vi "MGCC_StaEst_error_cal.vi"(8 "f_MGCC_StaEst_An":dbl[][](array[numeric]), 9 "f_MGCC_StaEst_Vn":dbl[][](array[numeric]), 10 "cluster":T1) -> (0 "output_An":dbl[][](array[numeric]), 1 "Ang Err":dbl[][](array[numeric]), 2 "Mag Err":dbl[][](array[numeric]), 3 "output_Vn":dbl[][](array[numeric]))   [LabVIEW 2016]
uses:
  MGCC_StaEst_global.vi
  Model Management/Global_MdlMgmt.vi
  Finite State Machine/Sub-VIs/MGCC_FntStaMach_gobal.vi
  <vilib>/imath/engines/lvmath2/RunTimeEngine/IndexRead/NIMS M(S,$).vi
  <instcachedir>/0/NIMS M(S,$)_F24F360562DE41D8BE234322A2E15C65.lvgen/NIMS M(S,$)_F24F360562DE41D8BE234322A2E15C65_000.vi
  <vilib>/imath/engines/lvmath2/RunTimeEngine/BuiltInFunctions/length/NIMS_length(GV).vi
  <instcachedir>/0/NIMS_length(GV)_08A3D13377FD4E4B96F5795FBF3698FA.lvgen/NIMS_length(GV)_08A3D13377FD4E4B96F5795FBF3698FA_000.vi
  <vilib>/imathl/engines/lvmath/Functions/Error Handling/Create Error.vi
  <vilib>/imath/engines/lvmath2/RunTimeEngine/RangeToken/NIMS_Range_R3 - Integer.vi
  <instcachedir>/0/NIMS_Range_R3 - Integer_A435E2FF893B4C718FD5055FE39FE2F6.lvgen/NIMS_Range_R3 - Integer_A435E2FF893B4C718FD5055FE39FE2F6_000.vi
  <vilib>/imath/engines/lvmath2/RunTimeEngine/CommandStatement/MC_CommandStatement_break.vi
  <vilib>/imath/engines/lvmath2/RunTimeEngine/IndexRead/NIMS M($,S).vi
  <instcachedir>/0/NIMS M($,S)_3E5749BBB62E49528D4765A77F1F6D98.lvgen/NIMS M($,S)_3E5749BBB62E49528D4765A77F1F6D98_000.vi
  <vilib>/imath/engines/lvmath2/RunTimeEngine/IndexRead/NIMS V(S).vi
  <instcachedir>/0/NIMS V(S)_0488751826AF41519A22953C041130DC.lvgen/NIMS V(S)_0488751826AF41519A22953C041130DC_000.vi
  <vilib>/imath/engines/lvmath2/RunTimeEngine/IndexReplace/NIMS M(S,S)=S.vi
  <instcachedir>/0/NIMS M(S,S)=S_98E40400474E4398B113AE20298B4F82.lvgen/NIMS M(S,S)=S_98E40400474E4398B113AE20298B4F82_000.vi
  <vilib>/imath/engines/lvmath2/RunTimeEngine/IndexRead/NIMS M(S,S).vi
  <instcachedir>/0/NIMS M(S,S)_AC51E74150A542F7991B9634C66F3096.lvgen/NIMS M(S,S)_AC51E74150A542F7991B9634C66F3096_000.vi
  <vilib>/imath/engines/lvmath2/RunTimeEngine/ErrorHandling/NIMS_Create Error From Enums.vi
  <vilib>/imath/engines/lvmath2/RunTimeSupport/NIMS_Error if Not Equal.vi
  <instcachedir>/0/NIMS_Error if Not Equal_43252A79AD05436189442EC0C5E5AB8A.lvgen/NIMS_Error if Not Equal_43252A79AD05436189442EC0C5E5AB8A_000.vi
  <vilib>/imath/engines/lvmath2/RunTimeEngine/IndexRead/NIMS M(S).vi
  <instcachedir>/0/NIMS M(S)_B826C018497E4940AE96BD27B540B6FB.lvgen/NIMS M(S)_B826C018497E4940AE96BD27B540B6FB_000.vi
  <vilib>/imath/engines/lvmath2/RunTimeEngine/IndexReplace/NIMS M(S,$)=V.vi
  <instcachedir>/0/NIMS M(S,$)=V_BCCFA522A894489B8FA760383D74A164.lvgen/NIMS M(S,$)=V_BCCFA522A894489B8FA760383D74A164_000.vi
  <vilib>/imath/engines/lvmath2/RunTimeEngine/NodeEndStatement/NIMS_NodeEndStatement_Output.vi
  <instcachedir>/0/NIMS_NodeEndStatement_Output_53EC0D466D134D7ABD903AC30B43404B.lvgen/NIMS_NodeEndStatement_Output_53EC0D466D134D7ABD903AC30B43404B_002.vi
  <vilib>/imath/engines/lvmath2/RunTimeEngine/ErrorHandling/NIMS_Finalize Error.vi
panel:
  out "array w/ subset deleted":dbl[](array[numeric])
  out "error out":errorcluster
  out "f_MGCC_OnliTopoIden_EnergizedMatrix 2":dbl[](array[numeric])
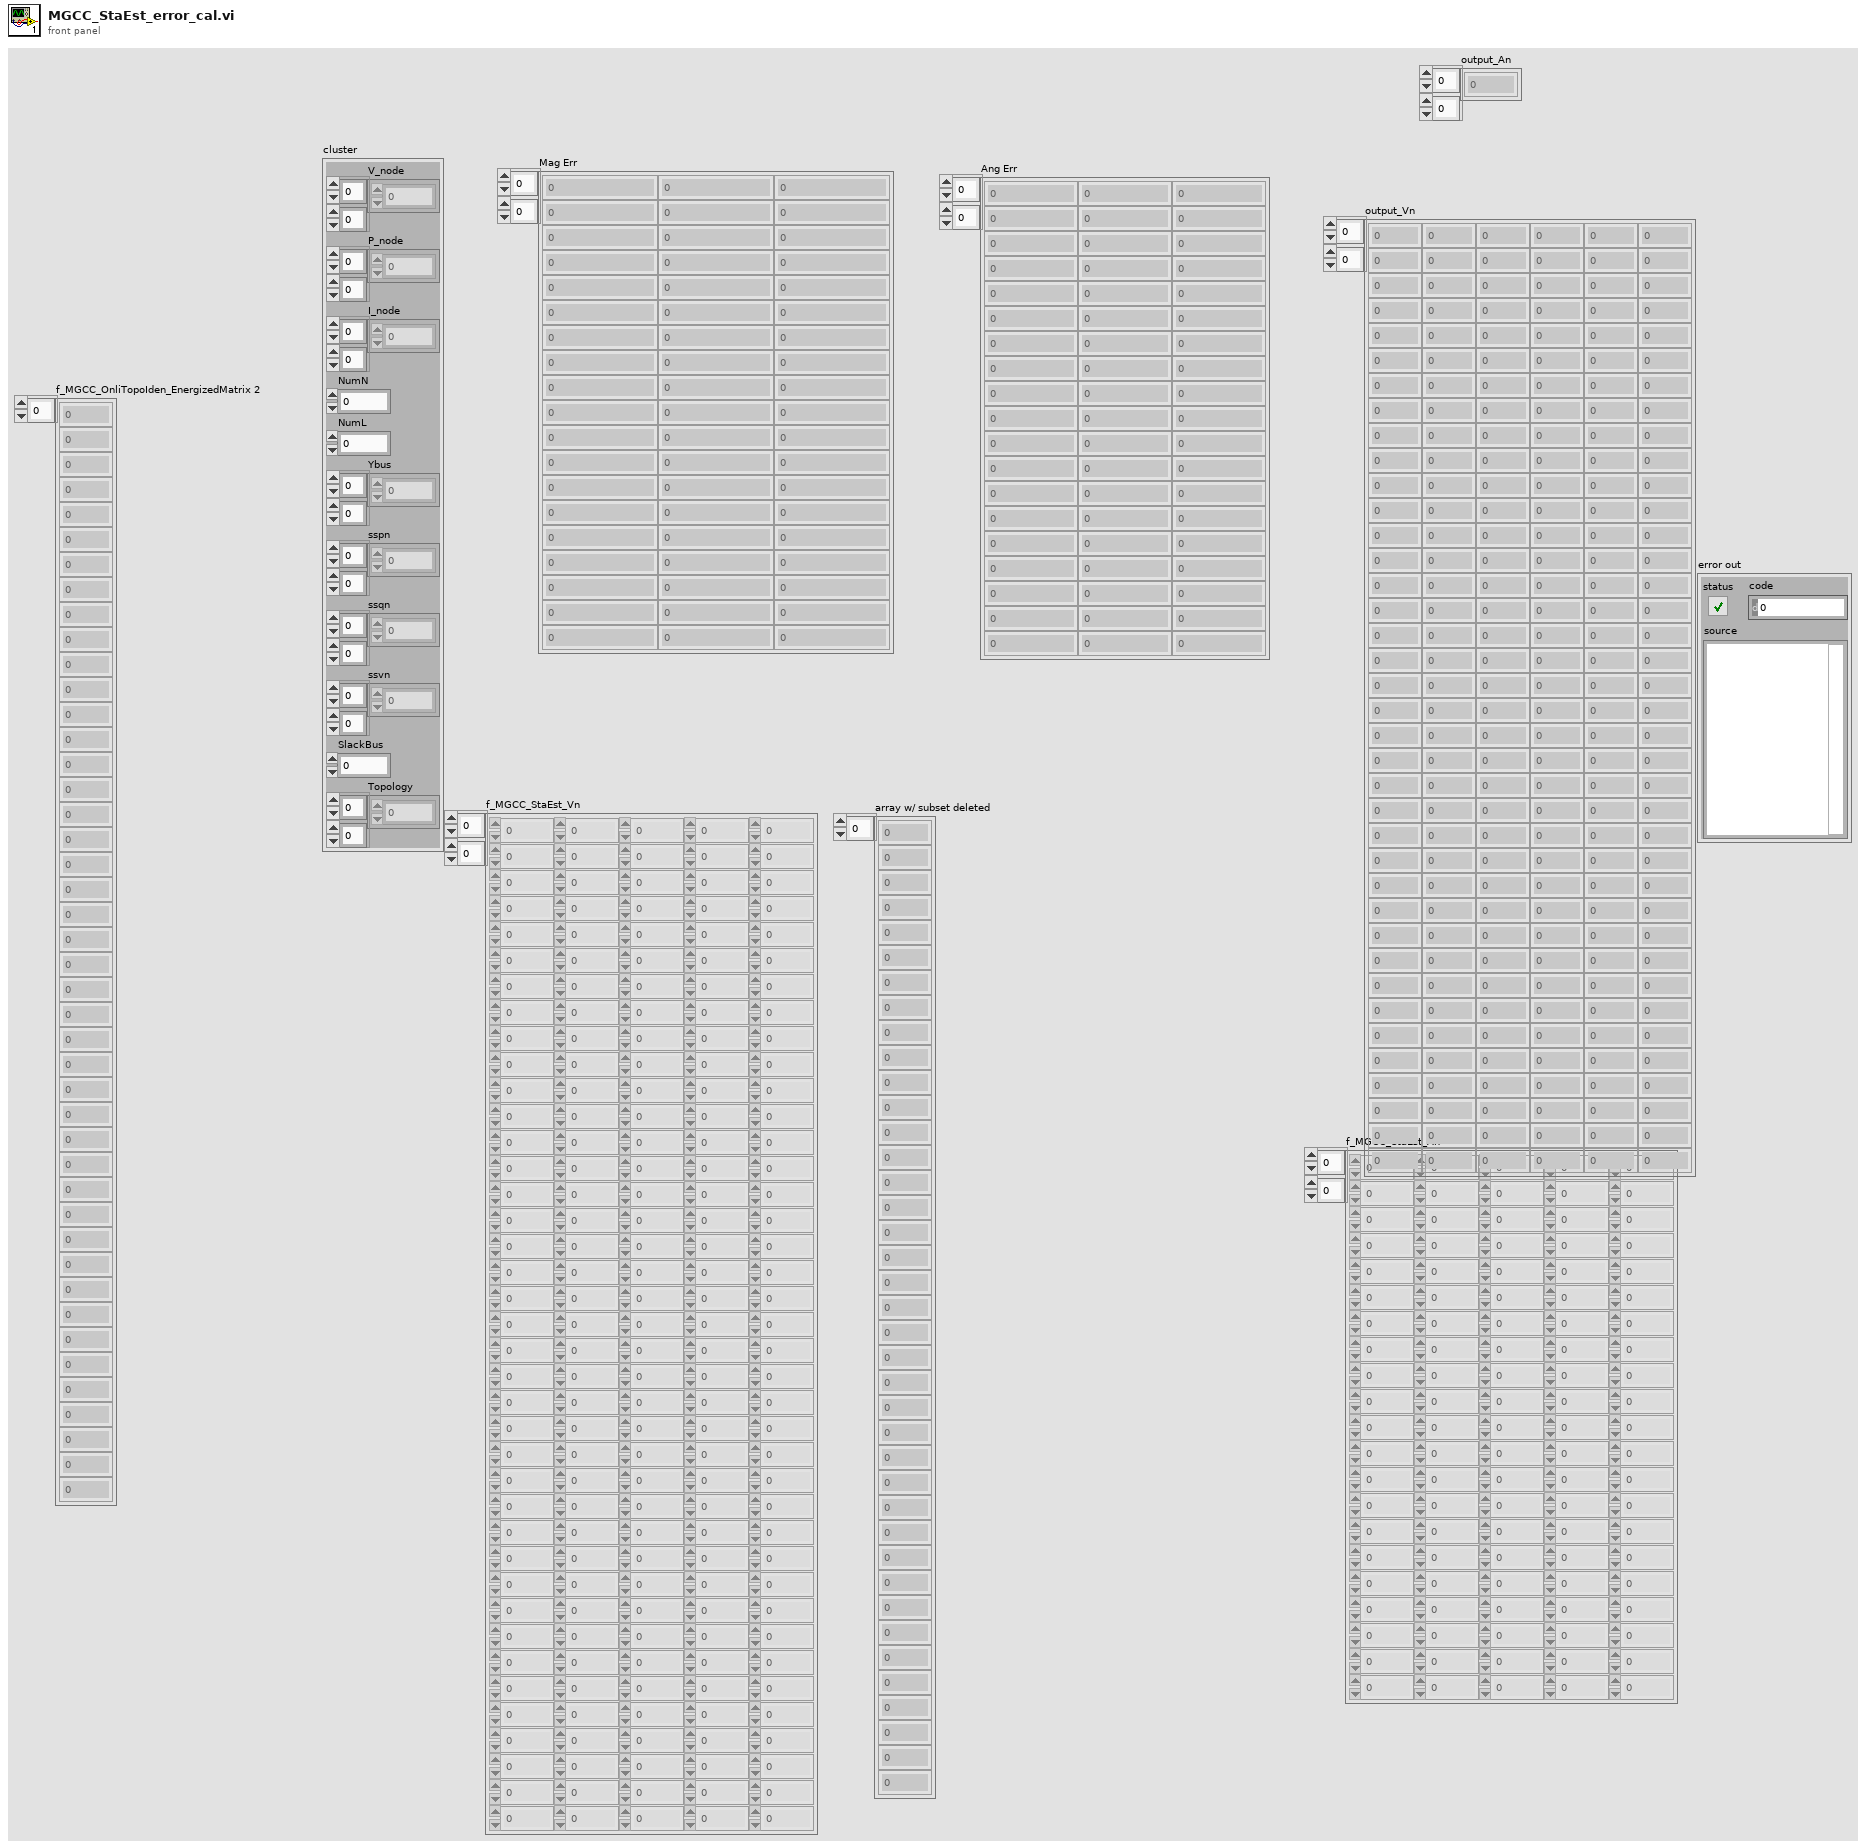
[diagram p1: front panel]
types:
  T1 = cluster{"V_node":cdb[][], "P_node":cdb[][], "I_node":cdb[][], "NumN":dbl, "NumL":dbl, "Ybus":cdb[][], "sspn":dbl[][], "ssqn":dbl[][], "ssvn":dbl[][], "SlackBus":dbl, "Topology":dbl[][]}
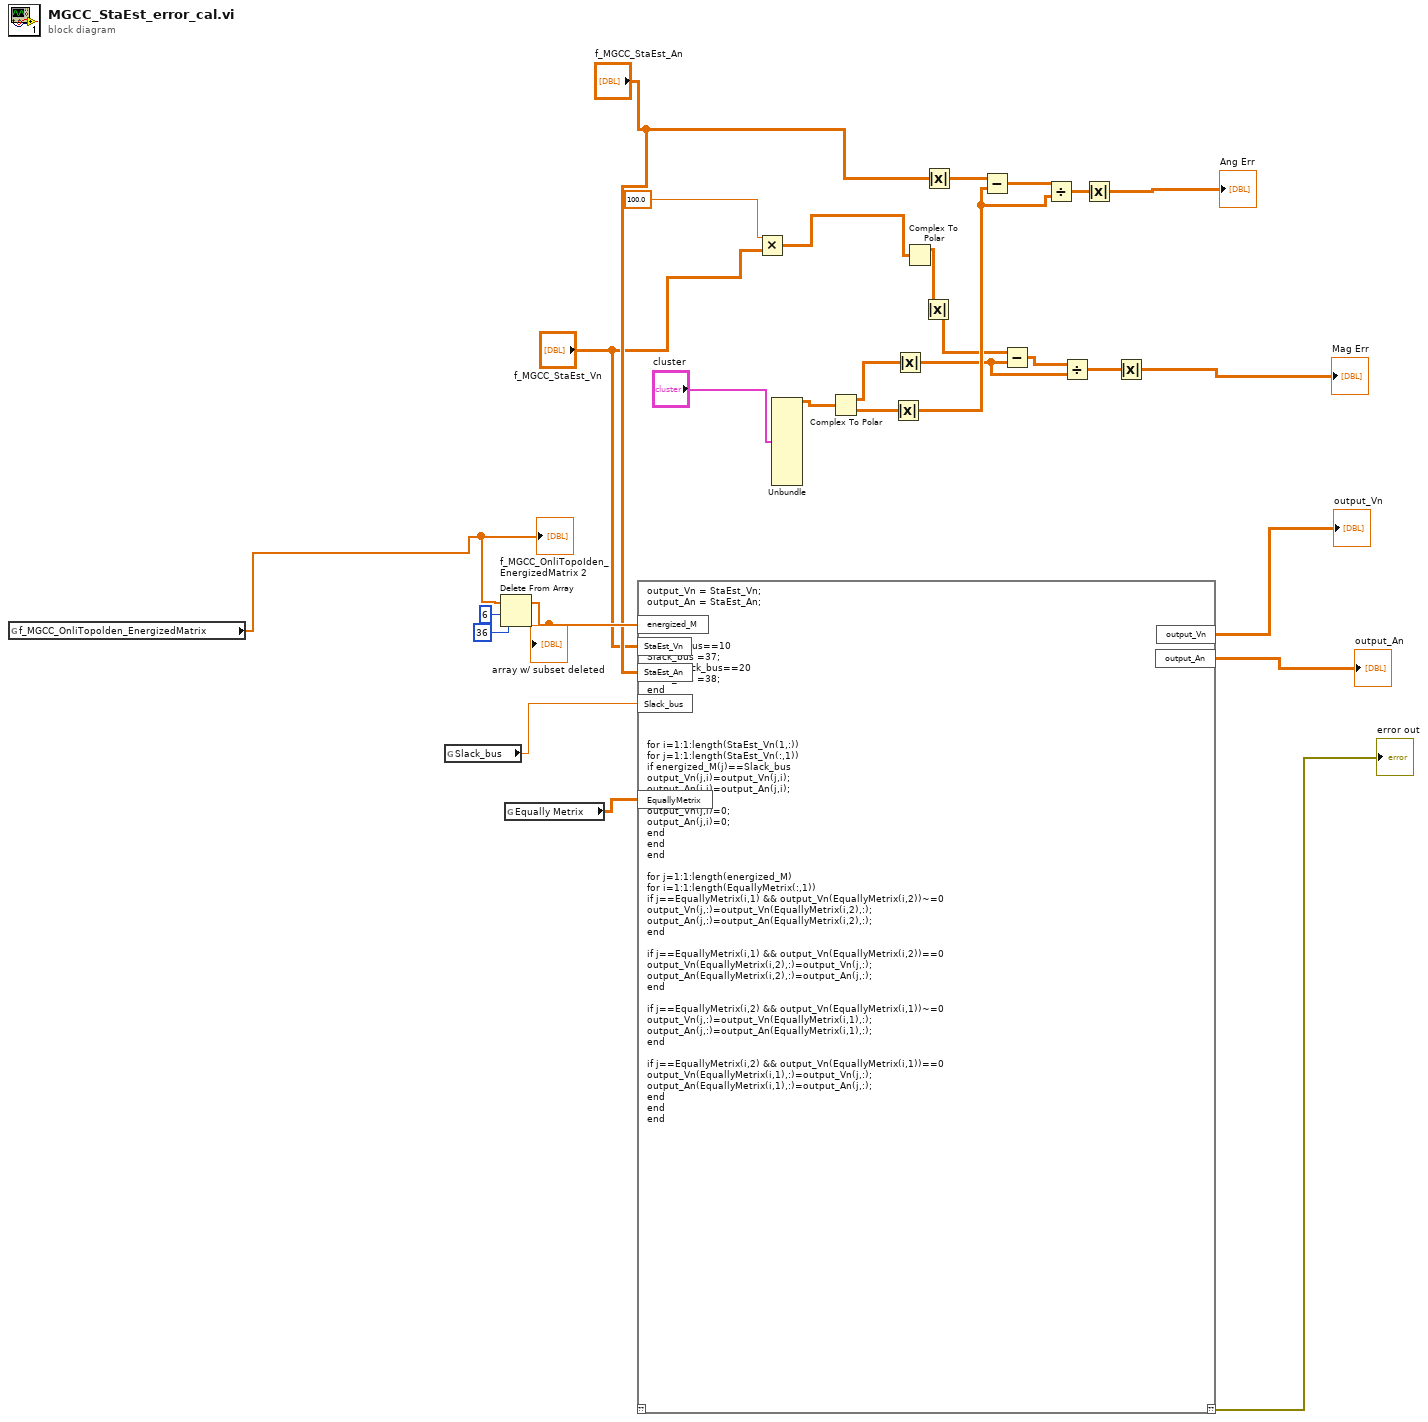
[diagram p0: block diagram]
diagram:
  n1 = global read "MGCC_FntStaMach_gobal.vi" "f_MGCC_OnliTopolden_EnergizedMatrix"() -> (w1:dbl[])
  "f_MGCC_OnliTopoIden_EnergizedMatrix 2" <- w1
  n2 = global read "MGCC_StaEst_global.vi" "Slack_bus"() -> (w3:dbl)
  n3 = Delete From Array(array=w1, length=6, index=36) -> (array with subset deleted=w9:dbl[])  [unwired: 1 out]
  "array w/ subset deleted" <- w9
  n4 = global read "Global_MdlMgmt.vi" "Equally Metrix"() -> (w2:dbl[][])
  n5 = mathscript code="output_Vn = StaEst_Vn;\noutput_An = StaEst_An;\n\n\n\nif Slack_bus==10\nSlack_bus =37;\nelseif Slack_bus==20\nSlack_bus =38;\nend\n\n\n\n\nfor i=1:1:length(StaEst_Vn(1,:))\nfor j=1:1:length(StaEst_Vn(:,1))\nif energized_M(j)==Slack_bus\noutput_Vn(j,i)=output_Vn(j,i);\noutput_An(j,i)=output_An(j,i);\nelse\noutput_Vn(j,i)=0;\noutput_An(j,i)=0;\nend\nend\nend\n\nfor j=1:1:length(energized_M)\nfor i=1:1:length(EquallyMetrix(:,1))\nif j==EquallyMetrix(i,1) && output_Vn(EquallyMetrix(i,2))~=0\noutput_Vn(j,:)=output_Vn(EquallyMetrix(i,2),:);\noutput_An(j,:)=output_An(EquallyMetrix(i,2),:);\nend\n\nif j==EquallyMetrix(i,1) && output_Vn(EquallyMetrix(i,2))==0\noutput_Vn(EquallyMetrix(i,2),:)=output_Vn(j,:);\noutput_An(EquallyMetrix(i,2),:)=output_An(j,:);\nend\n\nif j==EquallyMetrix(i,2) && output_Vn(EquallyMetrix(i,1))~=0\noutput_Vn(j,:)=output_Vn(EquallyMetrix(i,1),:);\noutput_An(j,:)=output_An(EquallyMetrix(i,1),:);\nend\n\nif j==EquallyMetrix(i,2) && output_Vn(EquallyMetrix(i,1))==0\noutput_Vn(EquallyMetrix(i,1),:)=output_Vn(j,:);\noutput_An(EquallyMetrix(i,1),:)=output_An(j,:);\nend\nend\nend"("energized_M"=w9, "StaEst_Vn"="f_MGCC_StaEst_Vn", "StaEst_An"="f_MGCC_StaEst_An", "Slack_bus"=w3, "EquallyMetrix"=w2) -> ("??"=→"error out":errorcluster, "output_Vn"=→"output_Vn":dbl[][], "output_An"=→"output_An":dbl[][])  [unwired: 1 in]
  n6 = Multiply(x=100.0, y="f_MGCC_StaEst_Vn") -> (x*y=w28:dbl[][])
  n7 = Unbundle("cluster") -> ("V_node"=w26:cdb[][])  [unwired: 10 out]
  n8 = Complex To Polar(r * e^(i*theta)=w26) -> (r=w23:dbl[][], theta=w20:dbl[][])
  n9 = Absolute Value(x=w20) -> (abs(x)=w17:dbl[][])
  n10 = Absolute Value(x=w23) -> (abs(x)=w15:dbl[][])
  n11 = Complex To Polar(r * e^(i*theta)=w28) -> (r=w25:dbl[][])  [unwired: 1 out]
  n12 = Absolute Value(x=w25) -> (abs(x)=w16:dbl[][])
  n13 = Absolute Value(x="f_MGCC_StaEst_An") -> (abs(x)=w18:dbl[][])
  n14 = Subtract(x=w18, y=w17) -> (x-y=w21:dbl[][])
  n15 = Subtract(x=w16, y=w15) -> (x-y=w24:dbl[][])
  n16 = Divide(x=w21, y=w17) -> (x/y=w19:dbl[][])
  n17 = Divide(x=w24, y=w15) -> (x/y=w22:dbl[][])
  n18 = Absolute Value(x=w19) -> (abs(x)=→"Ang Err":dbl[][])
  n19 = Absolute Value(x=w22) -> (abs(x)=→"Mag Err":dbl[][])
